vi "SubVI de Flip Flop D (3).vi"(11 "D0":bool) -> (3 "Q0*":bool)   [LabVIEW 2018]
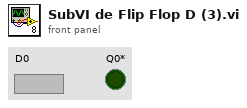
[diagram p1: front panel]
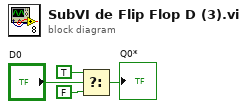
[diagram p0: block diagram]
diagram:
  n1 = Select(t=TRUE, s="D0", f=FALSE) -> (s? t:f=→"Q0*":bool)
